vi "Half_Adder.vi"() -> ()   [LabVIEW 2024]
panel:
  out "Carry":bool
  out "Sum":bool
  in  "y":bool
  in  "x":bool
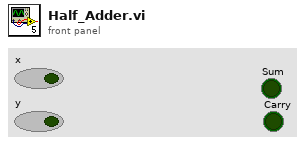
[diagram p1: front panel]
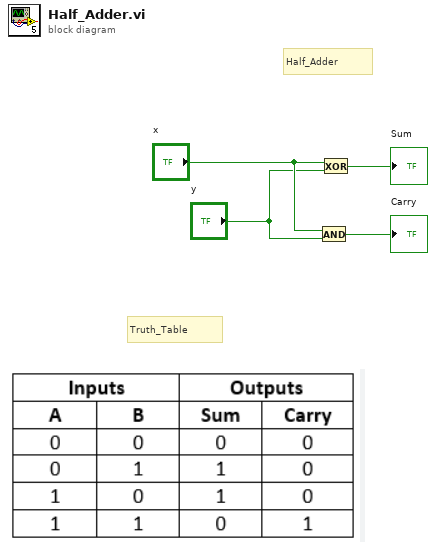
[diagram p0: block diagram]
diagram:
  # "Half_Adder"
  # "Truth_Table"
  n1 = And(x="x", y="y") -> (x .and. y?=→"Carry":bool)
  n2 = Exclusive Or(1:"y", 2:"x") -> (0:→"Sum":bool)
